vi "CommandPickup_FAST.vi"(9 "Gripper Value R":dbl, 10 "Gripper Value L":dbl, 11 "Elevator Value":dbl) -> (3 "appended array":cluster{"States":T1, "Close":dbl[]}[](array[cluster]))   [LabVIEW 2014, in "Elevator System.lvlib"]
uses:
  Elevator System.lvlib
  Typedef/ControllerStates.ctl
  Typedef/TeirNumber.ctl
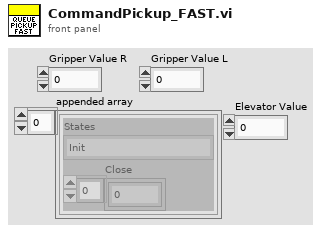
[diagram p1: front panel]
types:
  T1 = typedef "Elevator System.lvlib/ControllerStates.ctl" = enum16{"Init", "Set Elevator SP", "Set Gripper SP", "Wait For Elevator", "Wait For Gripper", "Wait For Elevator Fast", "Wait For Gripper Fast", "Disabled"}
  T2 = typedef "Elevator System.lvlib/TeirNumber.ctl" = enum16{"T1", "T2", "T3", "T4", "T5", "T6"}
  T3 = typedef "Elevator System.lvlib/GripperNotifierType.ctl" = cluster{"SP Left":dbl, "SP Right":dbl}
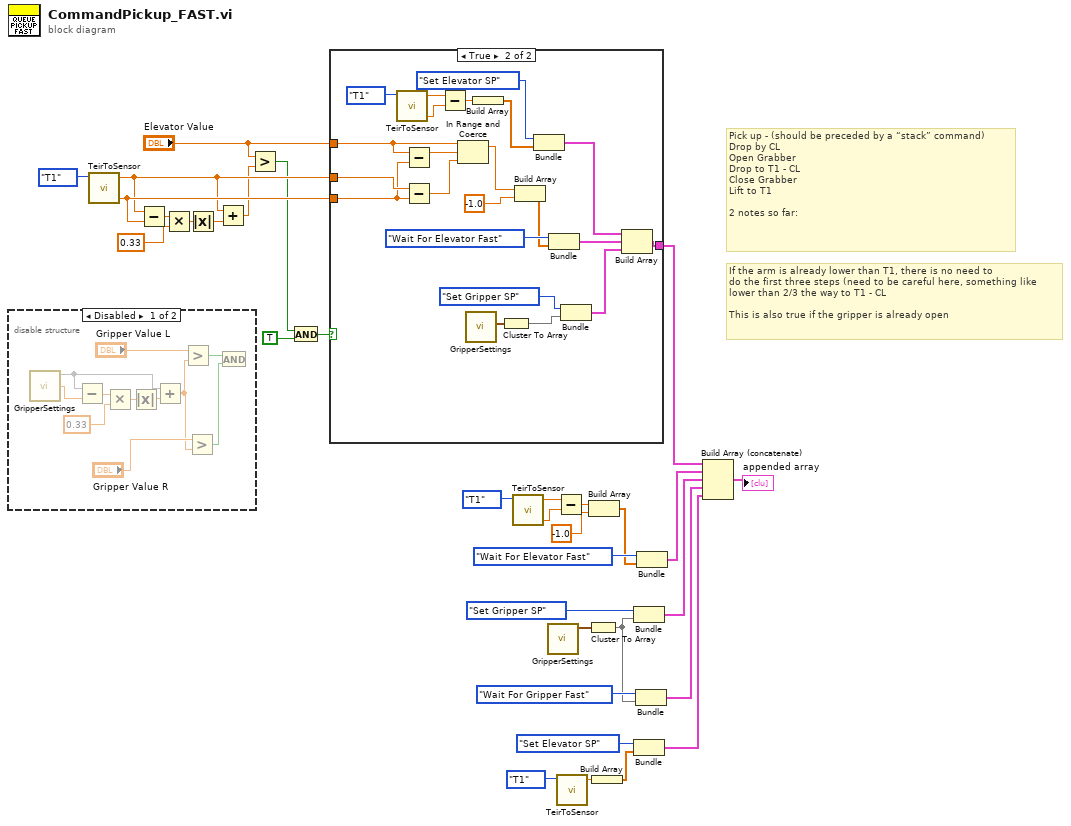
[diagram p0: block diagram]
diagram:
  # "If the arm is already lower than T1, there is no need to \ndo the first three steps (need to be careful here, something like \nlower than 2/3 the way to T1 - CL \n\nThis is also true if the gripper is already open"
  # "Pick up - (should be preceded by a “stack” command)\nDrop by CL\nOpen Grabber\nDrop to T1 - CL\nClose Grabber\nLift to T1\n\n2 notes so far:"
  n1 = disable-structure shown="Disabled" {
    frame Disabled {
      n2 = call "GripperSettings.vi"() -> ("Travel Detect"=w39:dbl, 8:w44)  [unwired: 3 in, 4 out]
      n3 = Subtract(x=w44, y=w39) -> (x-y=w40:dbl)
      n4 = Multiply(x=w40, y=0.33) -> (x*y=w42:dbl)
      n5 = Absolute Value(x=w42) -> (abs(x)=w43:dbl)
      n6 = Add(x=w44, y=w43) -> (x+y=w35:dbl)
      n7 = Greater?(x="Gripper Value L", y=w35) -> (0:w37:bool)
      n8 = Greater?(x="Gripper Value R", y=w35) -> (0:w34:bool)
      n9 = And(x=w37, y=w34) -> ()  [unwired: 1 out]
    }
    frame Enabled {
    }
  }
  n10 = call "TeirToSensor.vi"("Enum"=TeirNumber."T1") -> ("T1"=w16:dbl, "CL"=w20:dbl)  [unwired: 3 in, 3 out]
  n11 = Subtract(x=w16, y=w20) -> (x-y=w19:dbl)
  n12 = Multiply(x=w19, y=0.33) -> (x*y=w17:dbl)
  n13 = Absolute Value(x=w17) -> (abs(x)=w14:dbl)
  n14 = Add(x=w16, y=w14) -> (x+y=w15:dbl)
  n15 = Greater?(x="Elevator Value", y=w15) -> (0:w12:bool)
  n16 = And(x=w12, y=TRUE) -> (x .and. y?=w13:bool)
  n17 = case shown="True" w13 {
    tunnel: w16 -> [_ w64]
    tunnel: w20 -> [_ w63]
    tunnel: "Elevator Value" -> [_ w61]
    tunnel: [_ w58] -> w21
    frame False {
    }
    frame True {
      n18 = call "TeirToSensor.vi"("Enum"=TeirNumber."T1") -> ("T1"=w51:dbl, "CL"=w52:dbl)  [unwired: 3 in, 3 out]
      n19 = Subtract(x=w61, y=w63) -> (x-y=w65:dbl)
      n20 = Subtract(x=w64, y=w63) -> (x-y=w62:dbl)
      n21 = Subtract(x=w51, y=w52) -> (x-y=w49:dbl)
      n22 = In Range and Coerce(upper limit=w61, x=w65, lower limit=w62) -> (coerced(x)=w47:dbl)  [unwired: 1 out]
      n23 = call "GripperSettings.vi"() -> ("Open"=w56:T3)  [unwired: 5 in, 4 out]
      n24 = Build Array(w49) -> (w48:dbl[])
      n25 = Cluster To Array(cluster=w56) -> (array=w55:dbl[])
      n26 = Build Array(w47, -1.0 ("element")) -> (w46:dbl[])
      n27 = Bundle("States"=ControllerStates."Set Elevator SP", w48) -> (w60:cluster{"States":T1, dbl[]})  [unwired: 1 in]
      n28 = Bundle("States"=ControllerStates."Wait For Elevator Fast", w46) -> (w54:cluster{"States":T1, dbl[]})  [unwired: 1 in]
      n29 = Bundle("States"=ControllerStates."Set Gripper SP", "Open"=w55) -> (w59:cluster{"States":T1, "Open":dbl[]})  [unwired: 1 in]
      n30 = Build Array(w60, w54, w59) -> (w58:cluster{"States":T1, "Open":dbl[]}[])
    }
  }
  n31 = call "TeirToSensor.vi"("Enum"=TeirNumber."T1") -> ("T1"=w28:dbl, "CL"=w29:dbl)  [unwired: 3 in, 3 out]
  n32 = call "GripperSettings.vi"() -> ("Close"=w10:T3)  [unwired: 5 in, 4 out]
  n33 = Subtract(x=w28, y=w29) -> (x-y=w26:dbl)
  n34 = call "TeirToSensor.vi"("Enum"=TeirNumber."T1") -> ("T1"=w31:dbl)  [unwired: 3 in, 4 out]
  n35 = Cluster To Array(cluster=w10) -> (array=w6:dbl[])
  n36 = Build Array(w26, -1.0 ("element")) -> (w3:dbl[])
  n37 = Build Array(w31) -> (w9:dbl[])
  n38 = Bundle("States"=ControllerStates."Set Gripper SP", "Close"=w6) -> (w24:cluster{"States":T1, "Close":dbl[]})  [unwired: 1 in]
  n39 = Bundle("States"=ControllerStates."Set Elevator SP", w9) -> (w33:cluster{"States":T1, dbl[]})  [unwired: 1 in]
  n40 = Bundle("States"=ControllerStates."Wait For Gripper Fast", "Close"=w6) -> (w5:cluster{"States":T1, "Close":dbl[]})  [unwired: 1 in]
  n41 = Bundle("States"=ControllerStates."Wait For Elevator Fast", w3) -> (w2:cluster{"States":T1, dbl[]})  [unwired: 1 in]
  n42 = Build Array (concatenate)(w21, w2, w24, w5, w33) -> (→"appended array":cluster{"States":T1, "Close":dbl[]}[])
